vi "Relation Column Name.vi"(10 "From Mapping":T1, 11 "Reverse by Name":string) -> (2 "Column Name":string)   [LabVIEW 2020, in "Conditum SQLite.lvlib" / "SQLite.lvclass"]
uses:
  SQLite.lvclass
  <vilib>/IlluminatedG/IG Conditum Base/Conditum/Relation Mapping.ctl
  SQLite.lvclass/SQLite.ctl
  <vilib>/IlluminatedG/IG Conditum Base/Conditum/Conditum.lvlib
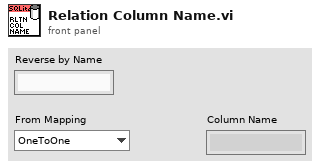
[diagram p1: front panel]
types:
  T1 = typedef "Conditum.lvlib/Relation Mapping.ctl" = enum16{"OneToOne", "OneToMany", "ManyToOne", "ManyToMany"}
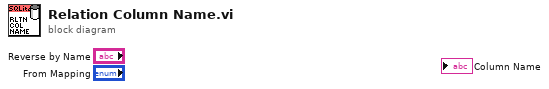
[diagram p0: block diagram]
diagram:
